vi "DiffDriveTrainSim_Execute.vi"(5 "LinearSystem_ID_DiffDrv_Model":T6={"TracWidth_M"=0.75, "WheelRadius_M"=26.0, "Gearing"=128.0, "Mass kg"=0.0, "MOI kgm2"=0.0, "DCMOTOR_TYPES"=enum."CIM", "Num Motors"=0} {"MOI kgm2" format="%#_13g"; "Mass kg" format="%#_13g"; "Gearing" format="%#_13g"; "WheelRadius_M" format="%#_13g"; "TracWidth_M" format="%#_13g"}, 6 "dT Sec":dbl=0.02, 7 "DiffDriveSim_Simulation _Params":T5, 8 "Initial Pose":T8={"TRANSLATION"={"X"=0.0, "Y"=0.0}, "ROTATION"={"VALUE"=0.0, "COS"=1.0, "SIN"=0.0}} {"ROTATION"."SIN" format="%13.4f"; "ROTATION"."COS" format="%13.4f"; "ROTATION"."VALUE" format="%13.4f"; "TRANSLATION"."Y" format="%14.3f"; "TRANSLATION"."X" format="%14.3f"}, 9 "BatteryVoltage":dbl=12.0, 10 "Right Motor Dmd":dbl=1.0, 11 "Left Motor Dmd":dbl=1.0) -> (0 "Error":bool, 3 "Outputs":dbl[](array[numeric]), 4 "out DiffDriveTrainSim":T1 {"m_Motor"."Jr_KgM2" format="%13.5p"; "m_Motor"."L_H" format="%13.5p"; "m_Motor"."Kt_NMPerAmp" format="%13.5p"; "m_Motor"."KvINV_RadPerSecPerVolt" format="%13.5p"; "m_Motor"."R_Ohms" format="%13.5p"; "m_Motor"."FreeSpeed_RadPerSec" format="%13.5p"; "m_Motor"."FreeCurrent_Amps" format="%13.5p"; "m_Motor"."StallCurrent_Amps" format="%13.5p"; "m_Motor"."StallTorque_NM" format="%13.5p"; "m_Motor"."nominalVoltage_Volts" format="%13.5p"})   [LabVIEW 2019, in "Trajectory_Library.lvlib"]
doc: "Single call LabVIEW function to simulate a Differential Drive Train system. \n\nThe diff drive simulation linear system contains:\n - states\n - X position meters \n - Y position meters - \n - heading radians \n - left velocity meter/sec- \n - right velocity meters/sec \n - left distance meters \n - right distance meters\n - inputs\n - left motor demand volts\n - right motor demand volts.\n - outputs\n - X position meters \n - Y position meters - \n - heading radians \n - left velocity meter/sec- \n - right velocity meters/sec \n - left distance meters \n - right distance meters\n\n \n\nInputs:\n - Linear System DiffDrv Model -- cluster -- Contains physical configuration for Diff Drive Train system.\n - Diff Drv Sim Simulation Params -- cluster -- Contains siulation configuration.\n - Initial Pose -- Pose2d -- Initial location of the drive train.\n - Left Motor Dmd (CO) -- double -- left motor demand value (+/- 1.0 )\n - Right Motor Dmd (CO) -- double -- right motor demand value (+/- 1.0 )\n - Battery Voltage -- double -- Current simulated battery voltage (Volts)\n - dT Sec -- double -- Update period (Seconds, Default: 0.02)\n\nOutputs:\n - Outputs -- double array -- Outputs. The index values are: \n 0 - X position meters \n 1 - Y position meters - \n 2 - heading radians \n 3 - left velocity meter/sec- \n 4 - right velocity meters/sec \n 5 - left distance meters \n 6 - right distance meters\n - Error -- boolean -- If TRUE an error occured.\n - outDiffDriveTrainSim -- cluster -- Current internal data cluster."
uses:
  Trajectory_Library.lvlib
  TypeDef/POSE2D.ctl
  TypeDef/TRANSLATION2D.ctl
  TypeDef/ROTATION2D.ctl
  TypeDef/DIFF_DRIVE_SIM_MODEL_PARAMS.CTL
  Enum/DCMOTOR_TYPES_ENUM.ctl
  TypeDef/DIFF_DRIVE_SIM_SIMULATION_PARAMS.ctl
  TypeDef/DIFF_DRIVE_TRAIN_SIM.ctl
  TypeDef/LINEAR_SYSTEM.ctl
  <vilib>/Analysis/Matrix/Datatypes/RealMatrix.ctl
  TypeDef/DCMOTOR.CTL
  MatBuilder_Create.vi
  DCMotor_GetCIM.vi
  DCMotor_GetAndymark9015.vi
  DCMotor_GetAndymarkRs775_125.vi
  DCMotor_GetBag.vi
  DCMotor_GetBanebotsRs550.vi
  DCMotor_GetBanebotsRs775.vi
  DCMotor_GetFalcon500.vi
  DCMotor_GetMiniCIM.vi
  DCMotor_GetNEO.vi
  DCMotor_GetNEO550.vi
  DCMotor_GetRomiBuiltIn.vi
  DCMotor_GetVex775Pro.vi
  DCMotor_GetAndymarkAM2235A.vi
  DCMotor_GetAndymarkAM3493.vi
  DCMotor_New.vi
  Units_RotationsPerMinuteToRadiansPerSecond.vi
  <vilib>/Analysis/Matrix/Numeric/Conversions/Matrix To Array - RM.vi
  <vilib>/Analysis/Matrix/NI_Matrix.lvlib
panel:
  # "<States, 1>"
  # "<Outputs, 1>"
  # "<Inputs, 1>"
  # "<Outputs, 1>"
  # "<States,States>"
  # "<States,Inputs>"
  # "<Outputs,States>"
  # "<Outputs,Inputs>"
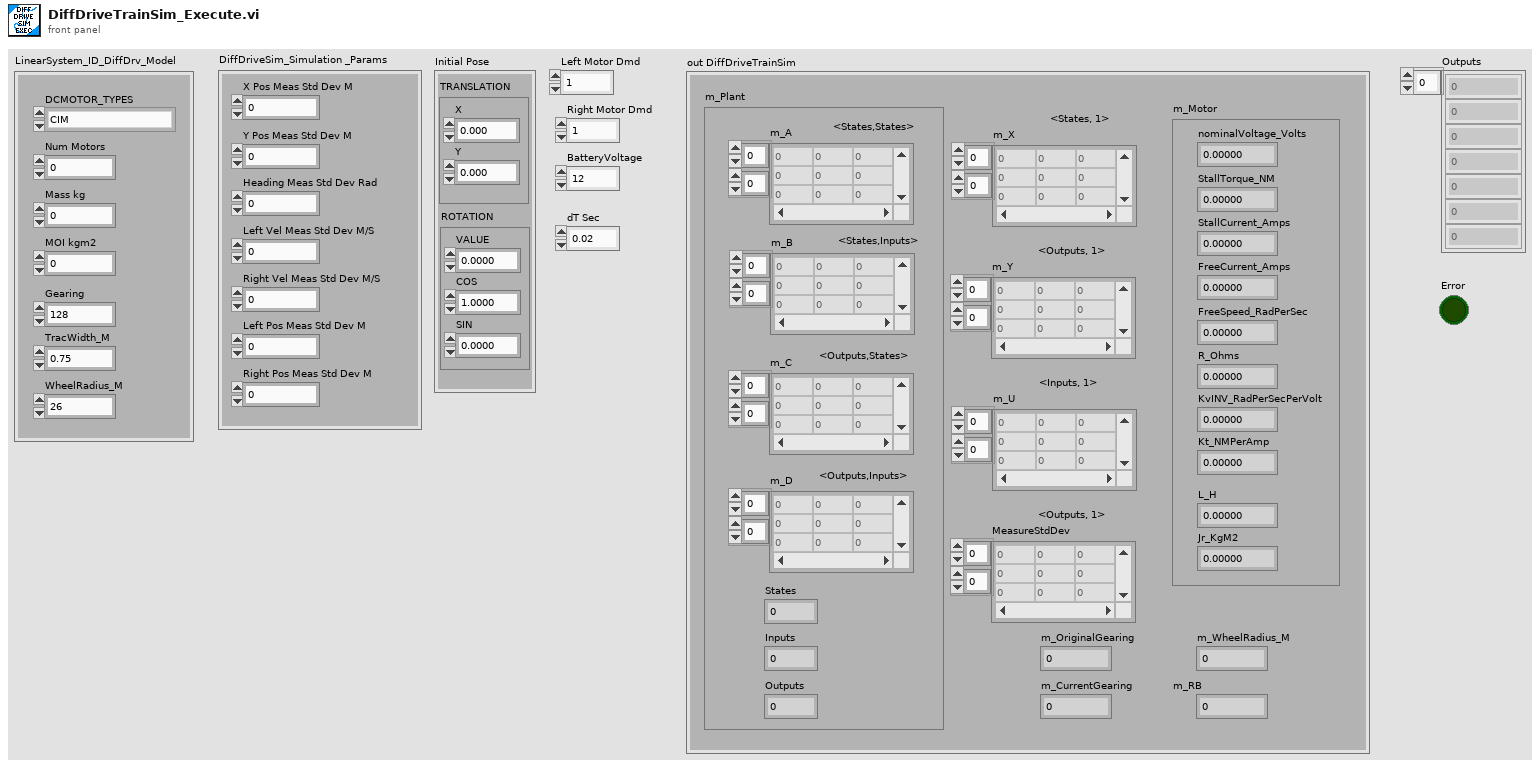
[diagram p1: front panel]
types:
  T1 = typedef "Trajectory_Library.lvlib/DIFF_DRIVE_TRAIN_SIM.ctl" = cluster{"m_Plant":T2, "m_X":T3, "m_Y":T3, "m_U":T3, "MeasureStdDev":T3, "m_Motor":T4, "m_OriginalGearing":dbl, "m_CurrentGearing":dbl, "m_WheelRadius_M":dbl, "m_RB":dbl}
  T2 = typedef "Trajectory_Library.lvlib/LINEAR_SYSTEM.ctl" = cluster{"m_A":T3, "m_B":T3, "m_C":T3, "m_D":T3, "States":i32, "Inputs":i32, "Outputs":i32}
  T3 = typedef "NI_Matrix.lvlib/RealMatrix.ctl" = dbl[][]
  T4 = typedef "Trajectory_Library.lvlib/DCMOTOR.CTL" = cluster{"nominalVoltage_Volts":dbl, "StallTorque_NM":dbl, "StallCurrent_Amps":dbl, "FreeCurrent_Amps":dbl, "FreeSpeed_RadPerSec":dbl, "R_Ohms":dbl, "KvINV_RadPerSecPerVolt":dbl, "Kt_NMPerAmp":dbl, "L_H":dbl, "Jr_KgM2":dbl}
  T5 = typedef "Trajectory_Library.lvlib/DIFF_DRIVE_SIM_SIMULATION_PARAMS.ctl" = cluster{"X Pos Meas Std Dev M":dbl, "Y Pos Meas Std Dev M":dbl, "Heading Meas Std Dev Rad":dbl, "Left Vel Meas Std Dev M/S":dbl, "Right Vel Meas Std Dev M/S":dbl, "Left Pos Meas Std Dev M":dbl, "Right Pos Meas Std Dev M":dbl}
  T6 = typedef "Trajectory_Library.lvlib/DIFF_DRIVE_SIM_MODEL_PARAMS.CTL" = cluster{"TracWidth_M":dbl, "WheelRadius_M":dbl, "Gearing":dbl, "Mass kg":dbl, "MOI kgm2":dbl, "DCMOTOR_TYPES":T7, "Num Motors":i32}
  T7 = typedef "Trajectory_Library.lvlib/DCMOTOR_TYPES_ENUM.ctl" = enum16{"CIM", "AndyMark 9015", "Andy Mark RS 775 125", "Bag", "BaneBots RS 550", "BaneBots RS 775", "Falcon 500", "Mini CIM", "NEO", "NEO 550", "Romi BuiltIn", "Vex 775 Pro", "Snow Blower AM 2235A", "Bosch Seat AM 3493"}
  T8 = typedef "Trajectory_Library.lvlib/POSE2D.ctl" = cluster{"TRANSLATION":T9, "ROTATION":T10}
  T9 = typedef "Trajectory_Library.lvlib/TRANSLATION2D.ctl" = cluster{"X":dbl, "Y":dbl}
  T10 = typedef "Trajectory_Library.lvlib/ROTATION2D.ctl" = cluster{"VALUE":dbl, "COS":dbl, "SIN":dbl}
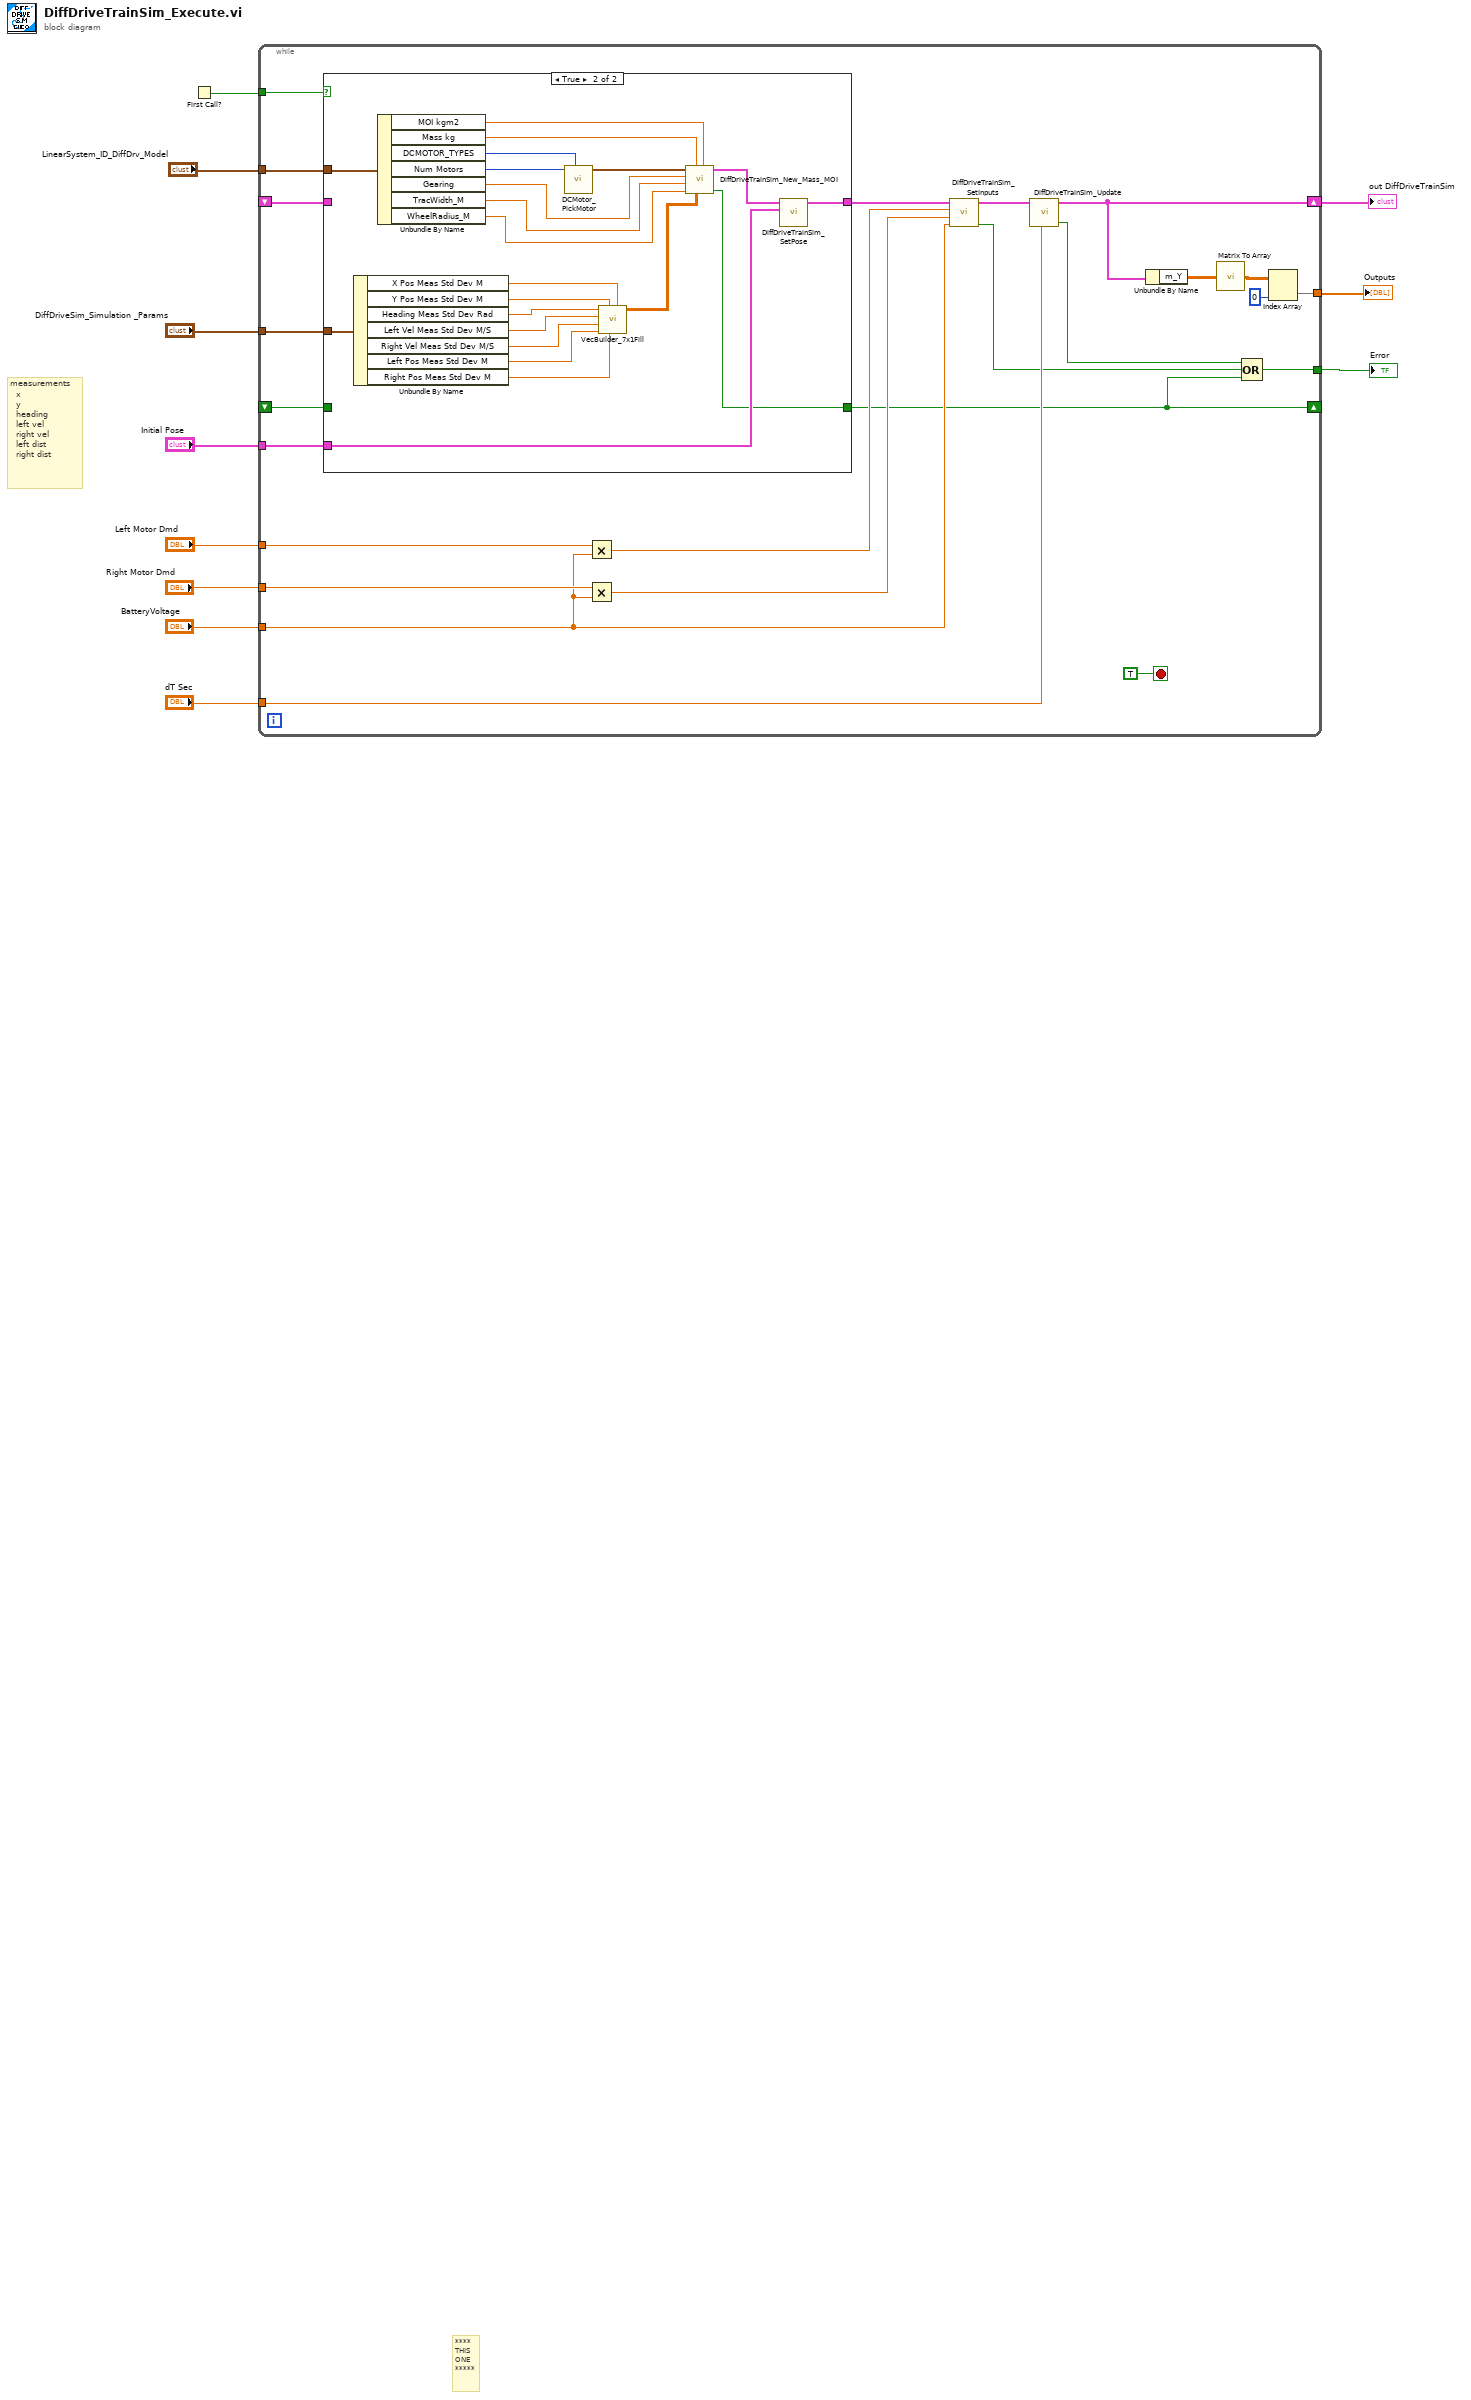
[diagram p0: block diagram]
diagram:
  # "measurements\n  x\n  y\n  heading\n  left vel\n  right vel\n  left dist\n  right dist"
  # "****\nTHIS\nONE\n*****"
  n1 = First Call?() -> (First Call?: T/F=w7:bool)
  n2 = while {
    shift-right: [w21] -> w3
    shift-left: _ -> [w32]
    tunnel: "Left Motor Dmd" -> [w29]
    tunnel: "Right Motor Dmd" -> [w28]
    tunnel: "BatteryVoltage" -> [w27]
    tunnel: "Initial Pose" -> [w26]
    tunnel: w7 -> [w25]
    tunnel: "LinearSystem_ID_DiffDrv_Model" -> [w24]
    tunnel: "DiffDriveSim_Simulation _Params" -> [w23]
    tunnel: "dT Sec" -> [w22]
    tunnel: [w17] -> w2
    tunnel: [w16] -> w1
    shift-right: [w13] -> _
    shift-left: _ -> [w12]
    stop <- TRUE stop-if-true
    n3 = case shown="True" w25 {
      tunnel: [w37 w59] -> w33
      tunnel: w32 -> [w37 _]
      tunnel: w26 -> [_ w58]
      tunnel: w24 -> [_ w57]
      tunnel: w23 -> [_ w47]
      tunnel: [w36 w38] -> w13
      tunnel: w12 -> [w36 _]
      frame False {
      }
      frame True {
        n4 = Unbundle By Name(w47) -> ("X Pos Meas Std Dev M"=w46:dbl, "Y Pos Meas Std Dev M"=w45:dbl, "Heading Meas Std Dev Rad"=w44:dbl, "Left Vel Meas Std Dev M/S"=w43:dbl, "Right Vel Meas Std Dev M/S"=w42:dbl, "Left Pos Meas Std Dev M"=w41:dbl, "Right Pos Meas Std Dev M"=w40:dbl)
        n5 = Unbundle By Name(w57) -> ("MOI kgm2"=w55:dbl, "Mass kg"=w54:dbl, "DCMOTOR_TYPES"=w53:T7, "Num Motors"=w52:i32, "Gearing"=w50:dbl, "TracWidth_M"=w49:dbl, "WheelRadius_M"=w48:dbl)
        n6 = call "DCMotor_PickMotor.vi"("DCMOTOR_TYPES"=w53, "Num Motors"=w52) -> ("DCMOTOR"=w51:T4)  [unwired: 9 in]
        n7 = call "VecBuilder_7x1Fill.vi"("R0"=w46, "R6"=w40, "R1"=w45, "R5"=w41, "R4"=w42, "R3"=w43, "R2"=w44) -> ("output matrix"=w39:T3)  [unwired: 4 in]
        n8 = call "DiffDriveTrainSim_New_Mass_MOI.vi"("j_KgM2"=w55, "MeasurementStdDev"=w39, "Mass_Kg"=w54, "WheelRadius_M"=w48, "TrackWidth_M"=w49, "Gearing"=w50, "DriveMotor"=w51) -> ("Size Coerced"=w38:bool, "DiffDriveTrainSim"=w56:T1)  [unwired: 3 in]
        n9 = call "DiffDriveTrainSim_SetPose.vi"("Pose"=w58, "in DiffDriveTrainSim"=w56) -> ("out DiffDriveTrainSim"=w59:T1)  [unwired: 9 in]
      }
    }
    n10 = Multiply(x=w29, y=w27) -> (x*y=w31:dbl)
    n11 = Multiply(x=w28, y=w27) -> (x*y=w30:dbl)
    n12 = call "DiffDriveTrainSim_SetInputs.vi"("BatteryVoltage"=w27, "Right_Volts"=w30, "Left_Volts"=w31, "in DiffDriveTrainSim"=w33) -> ("Size Coerced"=w14:bool, "out DiffDriveTrainSim"=w35:T1)  [unwired: 6 in]
    n13 = call "DiffDriveTrainSim_Update.vi"("dT_Seconds"=w22, "in DiffDriveTrainSim"=w35) -> ("Error"=w15:bool, "out DiffDriveTrainSim"=w21:T1)  [unwired: 8 in]
    n14 = Unbundle By Name(w21) -> ("m_Y"=w20:T3)
    n15 = call-poly <vilib>:"Matrix To Array.vi"("Real Matrix"=w20) -> ("Real 2D Array"=w19:dbl[][])
    n16 = Compound Arithmetic op=OR(w15, w14, w13) -> (w16:bool)
    n17 = Index Array(array=w19, index (col)=0 ("disabled index (col)")) -> (element=w17:dbl[])  [unwired: 1 in]
  }
  "out DiffDriveTrainSim" <- w3
  "Outputs" <- w2
  "Error" <- w1
